vi "3.2.vi"(1 "B":dbl, 2 "功能选择":enum16{"相除", "相乘", "相减", "相加"}(ring), 3 "A":dbl) -> (0 "Result":dbl)   [LabVIEW 2017]
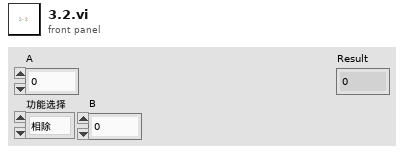
[diagram p1: front panel]
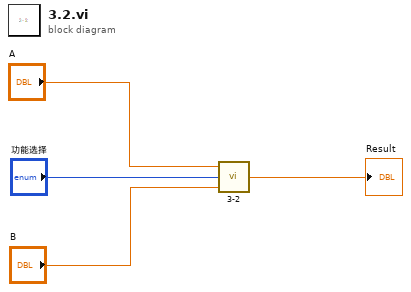
[diagram p0: block diagram]
diagram:
  n1 = call "3-2.vi"("B"="B", "功能选择"="功能选择", "A"="A") -> ("Result"=→"Result":dbl)
